vi "AR Drone - Simple Video + Simple nav.vi"() -> ()   [LabVIEW 2014]
doc: "Very simple example showing how to use the base VIs to control the AR Drone and receive and display video data."
uses:
  AR Drone - Simple Video + Simple nav Folder/Control cluster.ctl
  <vilib>/LVH/AR Drone Toolkit/Decode NavData/Typedefs/NavData Demo.ctl
  Global.vi
  <vilib>/LVH/AR Drone Toolkit/AR Drone.lvlib
panel:
  in  "Tab Control 2":enum32{"Setup", "Debug&Test Info", "NavData"}(tab)
  in  "Setup Parameters":T1={"Drone IP address"="192.168.1.1", "Home IP address"="192.168.1.2", "Flight Mode"=enum."INDOOR MODE", "Mounted Hull"=enum."INDOOR HULL", "Video Camera"=1, "Max Altitude (m)"=3.0, "Max Pitch and Roll Angle (deg)"=8.0, "Max Vertical Speed (m/s)"=0.7, "Max Yaw Speed (deg/s)"=100.0} {"Video Camera" items=["Bottom Camera"=1, "Front Camera"=0, "Front in Bottom"=3, "Bottom in Front"=2]}
  in  "device ID":i32=3
  in  "Video Acquisition VI path":path=path "Video Processing.vi"
  out "ctr+nav 2":i32=2242
  in  "milliseconds to wait":u32=10
  out "Refesh Rate (ms)":u32=5
  out "Refesh Rate Video Loop (ms) 2":u32
  in  "video refresh (ms)":u32=40
  out "ctr+nav":errorcluster
  out "NavData Out 2":T2={"control state"=enum."TRANS_LANDING", "battery percentage"=55, "pitch (deg)"=-0.02, "roll (deg)"=0.087, "yaw (deg)"=91.646, "altitude (cm)"=0, "vx (cm/s)?"=0.0, "vy (cm/s)?"=0.0, "vz (cm/s)?"=0.0, "detection cam type"=3}
  out "Battery Remaining 2":dbl(slide)=55.0 scale=0.0..100.0
  out "Hover":bool
  out "Control Cluster":T3={"Roll"=0.0, "Pitch"=-0.10223389, "Vertical Speed"=0.0, "Yaw Speed"=0.0} {"Yaw Speed" scale=-1.0..1.0; "Vertical Speed" scale=-1.0..1.0; "Pitch" scale=-1.0..1.0; "Roll" scale=-1.0..1.0}
  out "error":bool
  out "Take off/Land":bool
  in  "Tab Control":T4(tab)
  out "B&W":T5(plugin-control)
  out "Raw":picture
  out "OF":T5(plugin-control)
  in  "Manual":bool=TRUE
  in  "stop":bool
  in  "Emergency Landing":bool
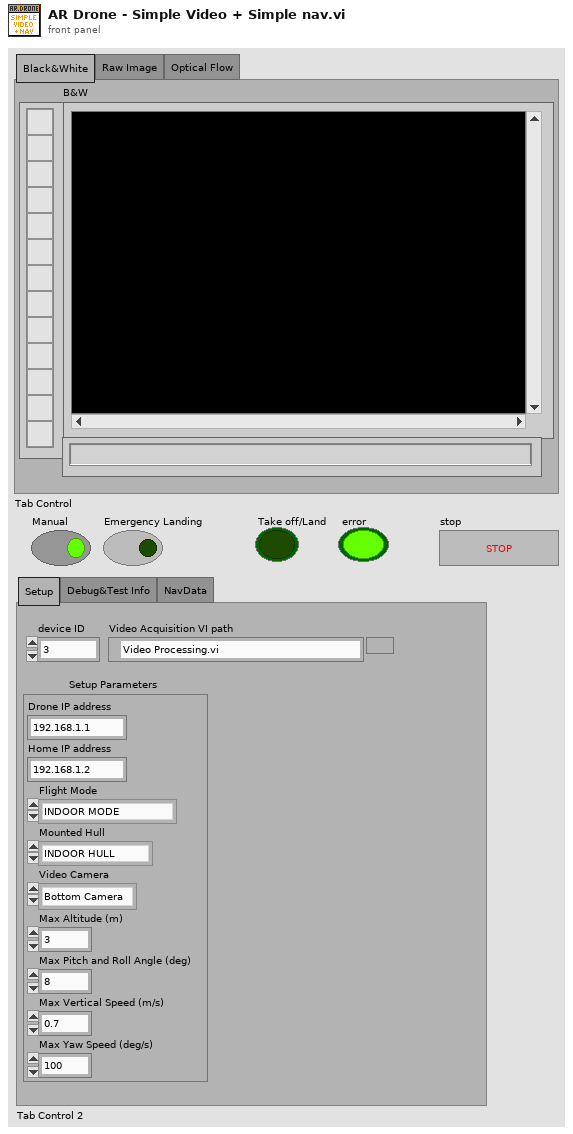
[diagram p1: front panel]
types:
  T1 = cluster{"Drone IP address":string, "Home IP address":string, "Flight Mode":enum8{"OUTDOOR MODE", "INDOOR MODE"}, "Mounted Hull":enum8{"OUTDOOR HULL", "INDOOR HULL"}, "Video Camera":u8, "Max Altitude (m)":sgl, "Max Pitch and Roll Angle (deg)":sgl, "Max Vertical Speed (m/s)":sgl, "Max Yaw Speed (deg/s)":sgl}
  T2 = typedef "AR Drone.lvlib/NavData Demo.ctl" = cluster{"control state":enum32{"DEFAULT", "INIT", "LANDING", "FLYING", "HOVERING", "TEST", "TRANS_TAKEOFF", "TRANS_GOTOFIX", "TRANS_LANDING"}, "battery percentage":u32, "pitch (deg)":sgl, "roll (deg)":sgl, "yaw (deg)":sgl, "altitude (cm)":u32, "vx (cm/s)?":sgl, "vy (cm/s)?":sgl, "vz (cm/s)?":sgl, "detection cam type":u32}
  T3 = typedef "Control cluster.ctl" = cluster{"Roll":sgl, "Pitch":sgl, "Vertical Speed":sgl, "Yaw Speed":sgl}
  T4 = enum32{"Black&White", "Raw Image", "Optical Flow"}
  T5 = typedef "IMAQ Image.ctl" = refnum<image>
  T6 = typedef "AR Drone.lvlib/AR Drone Resource.ctl" = cluster{"UDP Control Connection":refnum<k16>, "UDP NavData Connection":refnum<k16>, "UDP Video Connection (Drone 1.0)":refnum<k16>, "TCP Video Connection (Drone 2.0)":refnum<k5>, "TCP Control Port Connection":refnum<k5>, "Drone IP address":string, "Drone Command Port":u16, "Drone NavData Port":u16, "Drone Vid Stream Port":u16, "Drone TCP Control Port":u16, "Home IP address":string, "Home Command Port":u16, "Home NavData Port":u16, "Home Vid Stream Port":u16, "Drone Version":i32, "Drone Index":i32, "Command Sequence":i32}
  T7 = cluster{"Hover":bool, "Land/Take off":bool, "button 3":bool, "button 4":bool}
  T8 = cluster{"Roll":dbl, "Pitch":dbl, "Vertical Speed":dbl, "Yaw Speed":dbl}
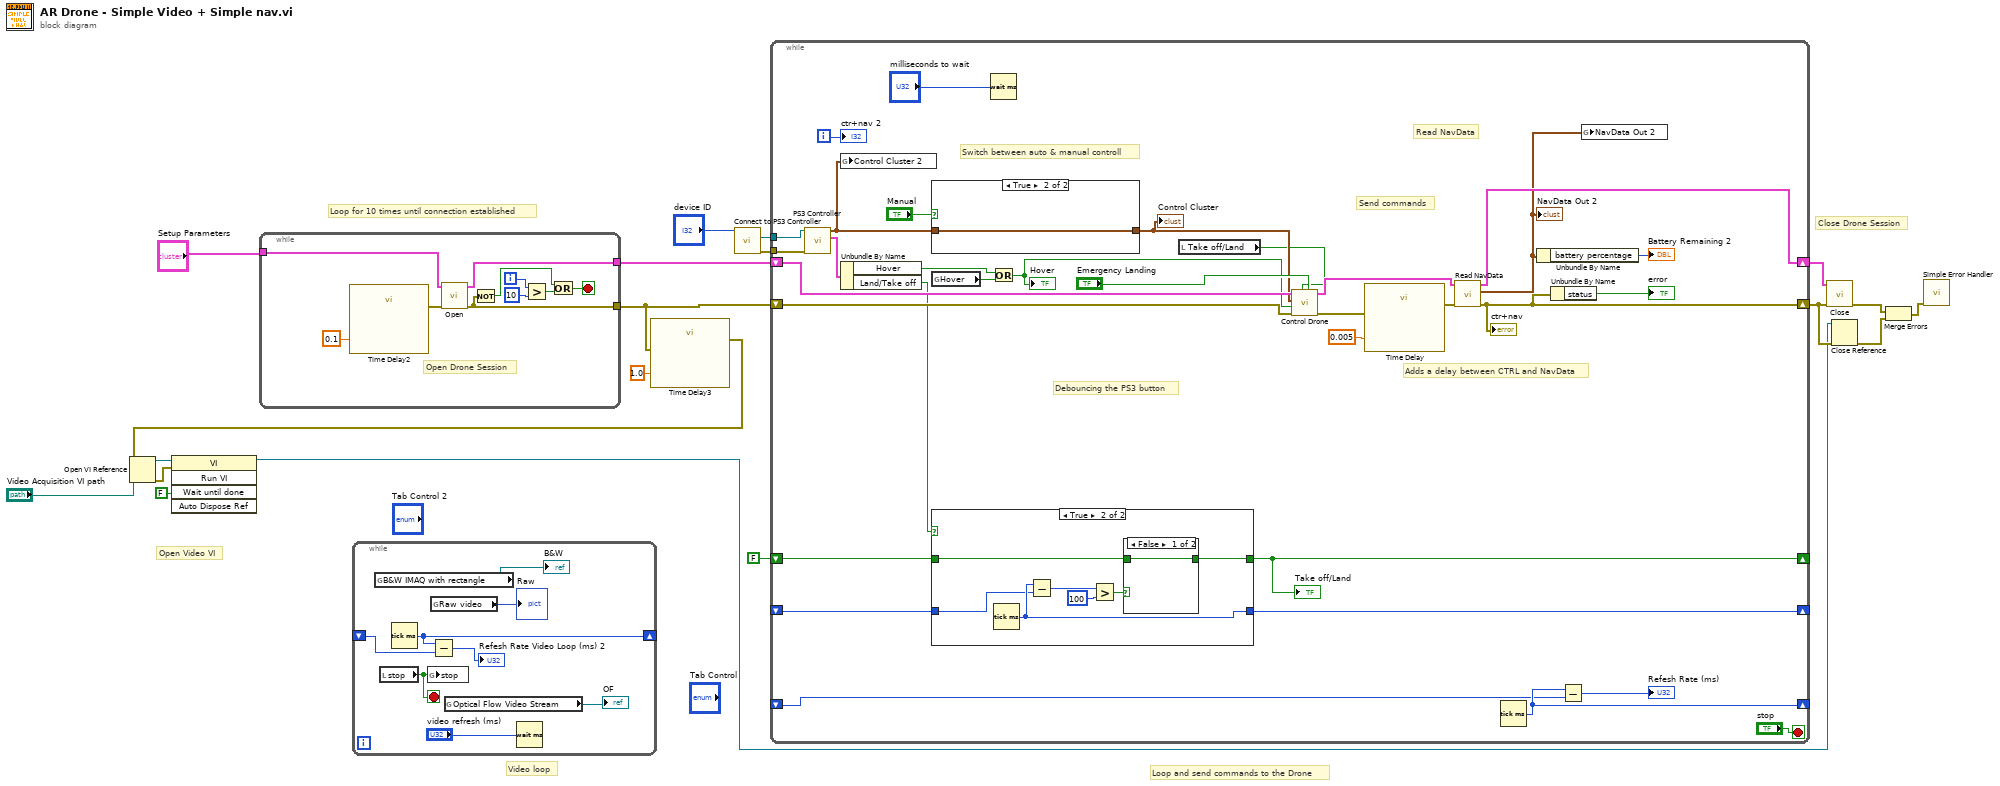
[diagram p0: block diagram]
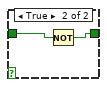
[diagram p3: hidden frame]
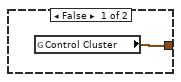
[diagram p4: hidden frame]
diagram:
  # "Open Video VI"
  # "Loop for 10 times until connection established"
  # "Video loop"
  # "Close Drone Session"
  # "Loop and send commands to the Drone"
  n1 = while {
    tunnel: [w21] -> w13
    tunnel: "Setup Parameters" -> [w29]
    tunnel: [w20] -> w5
    i -> [w25]
    stop <- w27 stop-if-true
    # "Open Drone Session"
    n2 = call "Time Delay2"("Delay Time (s)"=0.1) -> ("error out"=w22:errorcluster)  [unwired: 10 in]
    n3 = call <vilib>:"Open.vi"("error in (no error)"=w22, "Setup Parameters"=w29) -> ("error out"=w21:errorcluster, "AR Drone Resource"=w20:T6)  [unwired: 8 in]
    n4 = Not(x=w21) -> (.not. x?=w23:bool)
    n5 = Greater?(x=w25, y=10) -> (0:w26:bool)
    n6 = Or(x=w23, y=w26) -> (x .or. y?=w27:bool)
  }
  n7 = while {
    shift-right: [w35] -> _
    shift-left: _ -> [w34]
    stop <- w31 stop-if-true
    n8 = global read "Global.vi" "B&W IMAQ with rectangle"() -> (→"B&W":T5)
    n9 = local read "stop"() -> (w31:bool)
    n10 = Tick Count (ms)() -> (millisecond timer value=w35:u32)
    n11 = global write "Global.vi" "stop"(w31) -> ()
    n12 = global read "Global.vi" "Raw video"() -> (→"Raw":picture)
    n13 = Subtract(x=w35, y=w34) -> (x-y=→"Refesh Rate Video Loop (ms) 2":u32)
    n14 = global read "Global.vi" "Optical Flow Video Stream"() -> (→"OF":T5)
    n15 = Wait (ms)(milliseconds to wait="video refresh (ms)") -> ()  [unwired: 1 out]
  }
  n16 = call "Time Delay3"("error in (no error)"=w13, "Delay Time (s)"=1.0) -> ("error out"=w1:errorcluster)  [unwired: 9 in]
  n17 = Open VI Reference(vi path="Video Acquisition VI path", error in (no error)=w1) -> (vi reference=w9:refnum<vi>, error out=w7:errorcluster)  [unwired: 4 in]
  n18 = invoke class="VI" method="Run VI"(reference=w9, error in=w7, "Wait until done"=FALSE) -> (reference out=w10:refnum<vi>)  [unwired: 2 in, 4 out]
  n19 = call "Connect to PS3 Controller.vi"("device ID"="device ID") -> ("error out"=w16:errorcluster, "device ID 2"=w18:refnum<k1>)  [unwired: 7 in, 1 out]
  n20 = while {
    shift-right: [w39] -> w19
    shift-left: w5 -> [w67]
    shift-right: [w63] -> w11
    shift-left: w13 -> [w68]
    tunnel: w18 -> [w65]
    tunnel: w16 -> [w64]
    shift-right: [w55] -> _
    shift-left: _ -> [w54]
    shift-right: [w51] -> _
    shift-left: FALSE -> [w52]
    shift-right: [w50] -> _
    shift-left: _ -> [w49]
    i -> [w66]
    stop <- "stop" stop-if-true
    # "Read NavData"
    # "Send commands"
    # "Switch between auto & manual controll"
    # "Debouncing the PS3 button"
    # "Adds a delay between CTRL and NavData"
    n21 = call "PS3 Controller.vi"("error in (no error)"=w64, "device ID"=w65) -> ("Buttons control"=w62:T7, "Control cluster"=w47:T8)  [unwired: 6 in, 2 out]
    n22 = global write "Global.vi" "Control Cluster 2"(w47) -> ()
    n23 = Unbundle By Name(w62) -> ("Hover"=w58:bool, "Land/Take off"=w53:bool)
    n24 = case shown="True" "Manual" {
      tunnel: w47 -> [_ w84]
      tunnel: [w83 w84] -> w48
      frame False {
        n25 = global read "Global.vi" "Control Cluster"() -> (w83:T3)
      }
      frame True {
      }
    }
    "Control Cluster" <- w48
    n26 = global read "Global.vi" "Hover"() -> (w57:bool)
    n27 = case shown="True" w53 {
      tunnel: [w72 w73] -> w51
      tunnel: w52 -> [w72 w74]
      tunnel: [w71 w79] -> w50
      tunnel: w49 -> [w71 w78]
      frame False {
      }
      frame True {
        n28 = Tick Count (ms)() -> (millisecond timer value=w79:u32)
        n29 = Subtract(x=w79, y=w78) -> (x-y=w77:u32)
        n30 = Greater?(x=w77, y=u32 100) -> (0:w75:bool)
        n31 = case shown="False" w75 {
          tunnel: w74 -> [w80 w82]
          tunnel: [w80 w81] -> w73
          frame False {
          }
          frame True {
            n32 = Not(x=w82) -> (.not. x?=w81:bool)
          }
        }
      }
    }
    "Take off/Land" <- w51
    n33 = Wait (ms)(milliseconds to wait="milliseconds to wait") -> ()  [unwired: 1 out]
    n34 = Or(x=w58, y=w57) -> (x .or. y?=w56:bool)
    "Hover" <- w56
    n35 = local read "Take off/Land"() -> (w40:bool)
    n36 = call <vilib>:"Control Drone.vi"("Emergency Landing"="Emergency Landing", "Takeoff/Land"=w40, "error in (no error)"=w68, "Hover"=w56, "Control Cluster"=w48, "AR Drone Resource"=w67) -> ("error out"=w44:errorcluster, "AR Drone Resource Out"=w61:T6)  [unwired: 4 in]
    n37 = call "Time Delay"("error in (no error)"=w44, "Delay Time (s)"=0.005) -> ("error out"=w43:errorcluster)  [unwired: 9 in]
    n38 = call <vilib>:"Read NavData.vi"("error in (no error)"=w43, "AR Drone Resource"=w61) -> ("error out"=w63:errorcluster, "NavData Out"=w38:T2, "AR Drone Resource Out"=w39:T6)  [unwired: 7 in]
    "ctr+nav" <- w63
    "NavData Out 2" <- w38
    n39 = Tick Count (ms)() -> (millisecond timer value=w55:u32)
    n40 = Unbundle By Name(w38) -> ("battery percentage"=→"Battery Remaining 2":u32)
    n41 = Unbundle By Name(w63) -> ("status"=→"error":bool)
    n42 = Subtract(x=w55, y=w54) -> (x-y=→"Refesh Rate (ms)":u32)
    n43 = global write "Global.vi" "NavData Out 2"(w38) -> ()
    "ctr+nav 2" <- w66
  }
  n44 = call <vilib>:"Close.vi"("error in (no error)"=w11, "AR Drone Resource"=w19) -> ("error out"=w4:errorcluster)  [unwired: 9 in]
  n45 = Close Reference(reference=w10, error in (no error)=w11) -> (error out=w3:errorcluster)
  n46 = Merge Errors(w4, w3) -> (w2:errorcluster)
  n47 = call <vilib>:"Simple Error Handler.vi"("error in (no error)"=w2) -> ()  [unwired: 4 in, 5 out]
